vi "20211029_HW01.vi"() -> ()   [LabVIEW 2019]
panel:
  in  "Movev to End":bool
  in  "Del":bool
  in  "Add":bool
  in  "Listbox":i32(listbox)
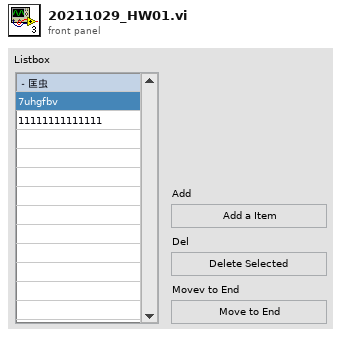
[diagram p1: front panel]
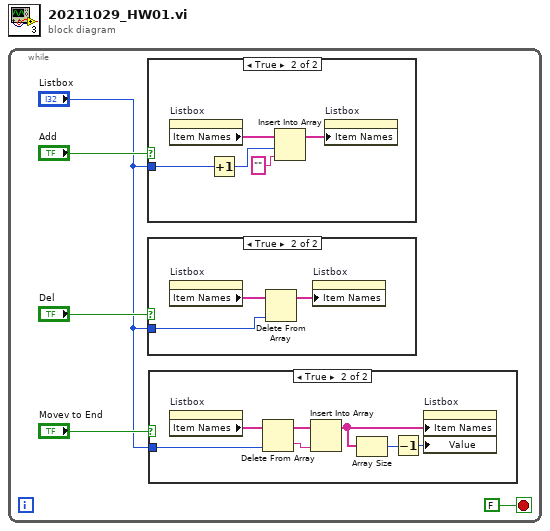
[diagram p0: block diagram]
diagram:
  n1 = while {
    stop <- FALSE stop-if-true
    n2 = case shown="True" "Add" {
      tunnel: "Listbox" -> [_ w9]
      frame False {
      }
      frame True {
        n3 = property on="Listbox" class="LstBox (strict)"() -> ("Item Names"=w13:string[])  [unwired: 2 in, 2 out]
        n4 = Increment(x=w9) -> (x+1=w10:i32)
        n5 = Insert Into Array(array=w13, index=w10, new element="" ("new element/subarray")) -> (w12:string[])
        n6 = property on="Listbox" class="LstBox (strict)"("Item Names"=w12) -> ()  [unwired: 2 in, 2 out]
      }
    }
    n7 = case shown="True" "Del" {
      tunnel: "Listbox" -> [_ w6]
      frame False {
      }
      frame True {
        n8 = property on="Listbox" class="LstBox (strict)"() -> ("Item Names"=w8:string[])  [unwired: 2 in, 2 out]
        n9 = Delete From Array(array=w8, index=w6) -> (array with subset deleted=w7:string[])  [unwired: 1 in, 1 out]
        n10 = property on="Listbox" class="LstBox (strict)"("Item Names"=w7) -> ()  [unwired: 2 in, 2 out]
      }
    }
    n11 = case shown="True" "Movev to End" {
      tunnel: "Listbox" -> [_ w19]
      frame False {
      }
      frame True {
        n12 = property on="Listbox" class="LstBox (strict)"() -> ("Item Names"=w20:string[])  [unwired: 2 in, 2 out]
        n13 = Delete From Array(array=w20, index=w19) -> (deleted portion=w17:string, array with subset deleted=w18:string[])  [unwired: 1 in]
        n14 = Insert Into Array(array=w18, new element=w17) -> (w16:string[])  [unwired: 1 in]
        n15 = Array Size(array=w16) -> (size(s)=w15:i32)
        n16 = Decrement(x=w15) -> (x-1=w14:i32)
        n17 = property on="Listbox" class="LstBox (strict)"("Item Names"=w16, "Value"=w14) -> ()  [unwired: 2 in, 2 out]
      }
    }
  }
